vi "Read Thermal Image Metadata.vi"(8 "error in (no error)":errorcluster, 11 "Optris PI in":refnum<class "Optris PI.lvclass">) -> (0 "error out":errorcluster, 2 "Thermal Image Metadata":u16[](array[numeric]), 3 "Optris PI out":refnum<class "Optris PI.lvclass">)   [LabVIEW 2018, in "Optris PI.lvlib" / "Optris PI.lvclass"]
uses:
  Optris PI.lvclass
  Optris PI.lvclass/Optris PI.ctl
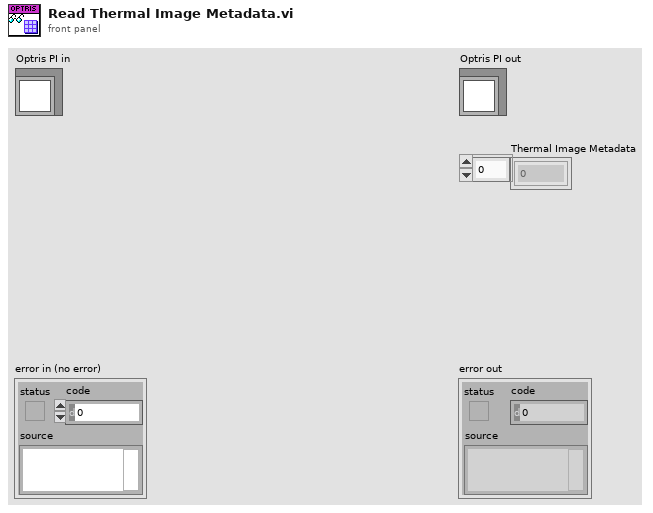
[diagram p1: front panel]
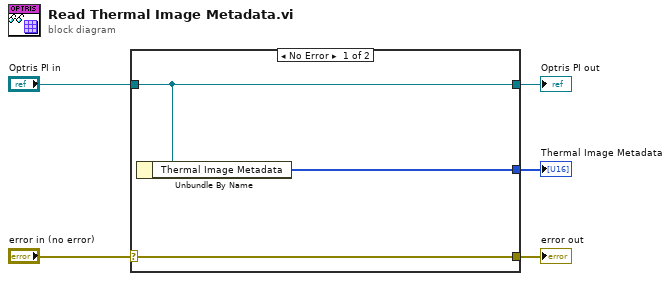
[diagram p0: block diagram]
diagram:
  n1 = case shown="No Error" "error in (no error)" {
    selector: "error in (no error)" -> [w8 w9]
    tunnel: [w8 w9] -> w4
    tunnel: [w7 w10] -> w2
    tunnel: "Optris PI in" -> [w7 w10]
    tunnel: [w6 _] -> w1
    frame No Error {
      n2 = Unbundle By Name(w7) -> ("Thermal Image Metadata"=w6:u16[])
    }
    frame Error {
    }
  }
  "error out" <- w4
  "Optris PI out" <- w2
  "Thermal Image Metadata" <- w1
